vi "Cluster Dialog_Select Unwired Terminals.vi"(9 "Select Unwired":bool, 10 "Display Items":T1[](array[typedef]), 11 "Tree Ref":refnum<vi>) -> (2 "Selected items":string[](array[string]), 3 "Tree Ref Out":refnum<vi>)   [LabVIEW 2023]
uses:
  cluster/Cluster Element Description.ctl
  <userlib>/_OpenG.lib/array/array.llb/openg_array.lvlib
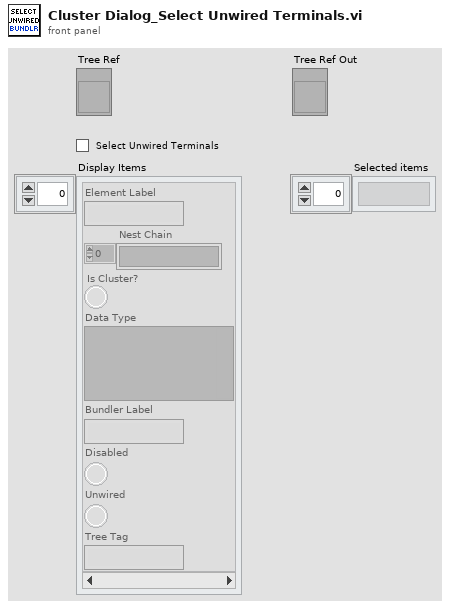
[diagram p1: front panel]
types:
  T1 = typedef "Cluster Element Description.ctl" = cluster{"Element Label":string, "Nest Chain":string[], "Is Cluster?":bool, "Data Type":variant, "Bundler Label":string, "Disabled":bool, "Unwired":bool, "Tree Tag":string}
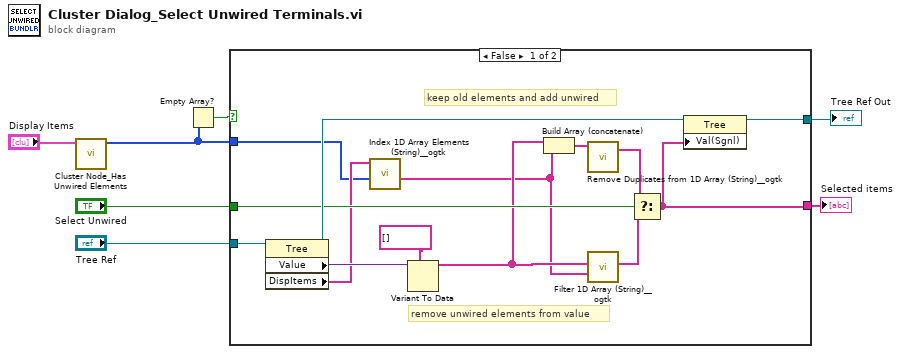
[diagram p0: block diagram]
diagram:
  n1 = call "Cluster Node_Has Unwired Elements.vi"("Display Items"="Display Items") -> ("Unwired Indicies"=w5:i32[])  [unwired: 9 in, 1 out]
  n2 = Empty Array?(array=w5) -> (empty?=w7:bool)
  n3 = case shown="False" w7 {
    tunnel: w5 -> [w12 _]
    tunnel: "Select Unwired" -> [w15 _]
    tunnel: "Tree Ref" -> [w18 w22]
    tunnel: [w9 _] -> w2
    tunnel: [w8 w22] -> w1
    frame False {
      # "keep old elements and add unwired"
      # "remove unwired elements from value"
      n4 = property class="Tree"(reference=w18) -> (reference out=w20:refnum<vi>, "Value"=w21:variant, "DispItems"=w13:string[])  [unwired: 1 in, 1 out]
      n5 = call <userlib>:"Index 1D Array Elements (String)__ogtk.vi"("indices"=w12, "array"=w13) -> ("elements"=w10:string[])  [unwired: 9 in]
      n6 = Variant To Data(type=string[] [] ("All Tags"), Variant=w21) -> (data=w11:string[])  [unwired: 1 in, 1 out]
      n7 = Build Array (concatenate)(w11, w10) -> (w17:string[])
      n8 = call <userlib>:"Remove Duplicates from 1D Array (String)__ogtk.vi"("Input Array"=w17) -> ("Output Array"=w16:string[])  [unwired: 1 out]
      n9 = call <userlib>:"Filter 1D Array (String)__ogtk.vi"("items to filter"=w10, "array"=w11) -> ("filtered array"=w19:string[])  [unwired: 4 in, 1 out]
      n10 = Select(t=w16, s=w15, f=w19) -> (s? t:f=w9:string[])
      n11 = property class="Tree"(reference=w20, "Val(Sgnl)"=w9) -> (reference out=w8:refnum<vi>)  [unwired: 1 in, 1 out]
    }
    frame True {
    }
  }
  "Selected items" <- w2
  "Tree Ref Out" <- w1
